vi "Sig2MS Process.vi"(5 "SigProc":bool, 6 "error in (no error)":errorcluster, 7 "Index":i32=-1, 8 "signal in":waveform(sgl), 9 "SkipIon":bool) -> (0 "error out":errorcluster, 1 "Ionisation signal out":waveform(sgl)[](array[waveform]), 2 "spectraData":waveform(sgl)[](array[waveform]), 4 "signalDataAttr":T1)   [LabVIEW 2018]
uses:
  Sig2MS.lvclass
  ctl/signalDataAttr.ctl
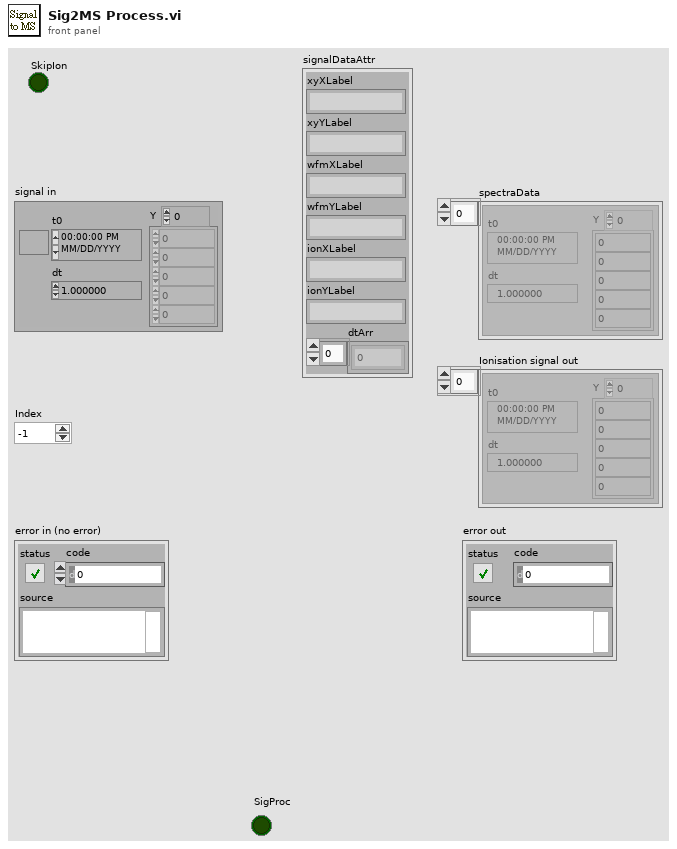
[diagram p1: front panel]
types:
  T1 = typedef "signalDataAttr.ctl" = cluster{"xyXLabel":string, "xyYLabel":string, "wfmXLabel":string, "wfmYLabel":string, "ionXLabel":string, "ionYLabel":string, "dtArr":dbl[]}
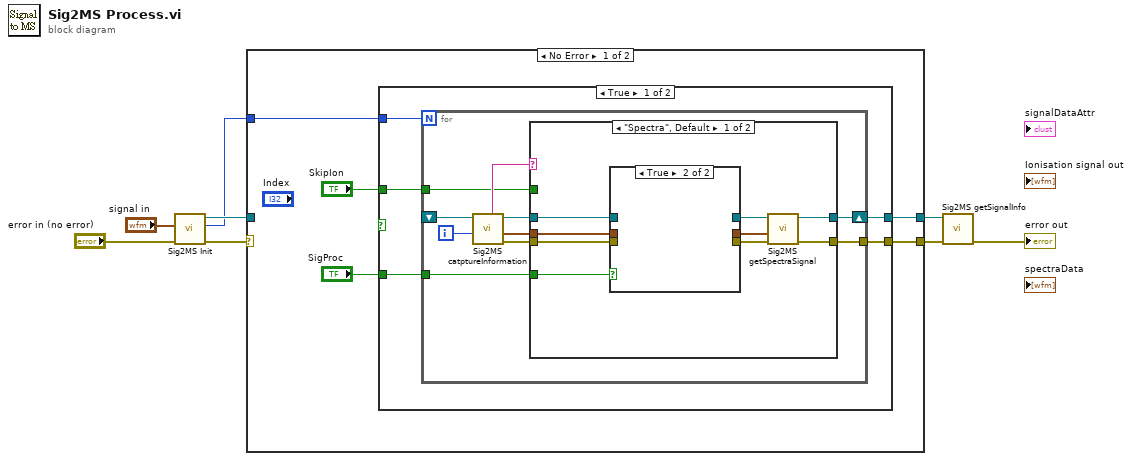
[diagram p0: block diagram]
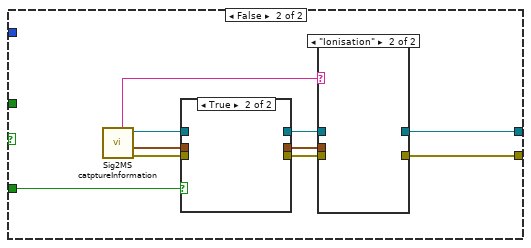
[diagram p5: hidden frame]
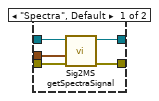
[diagram p7: hidden frame]
diagram:
  n1 = call "Sig2MS Init.vi"("error in (no error)"="error in (no error)", "signal in"="signal in") -> ("error out"=w5:errorcluster, "Size"=w2:i32, "Sig2MS out"=w6:refnum<class "Sig2MS.lvclass">)  [unwired: 7 in]
  n2 = case shown="No Error" w5 {
    selector: w5 -> [_ w68]
    tunnel: w6 -> [_ w69]
    tunnel: w2 -> [w13 _]
    tunnel: [w11 w68] -> w3
    tunnel: [w10 w69] -> w4
    frame No Error {
      n3 = case shown="True" {
        selector: _ -> [_ _]
        tunnel: w13 -> [w17 _]
        tunnel: "SigProc" -> [w18 w59]
        tunnel: [w16 w58] -> w11
        tunnel: [w15 w52] -> w10
        tunnel: "SkipIon" -> [w14 _]
        frame True {
          n4 = for {
            N: w17 -> [_]
            tunnel: w18 -> [w20]
            shift-right: [w27] -> w15
            shift-left: _ -> [w28]
            tunnel: [w26] -> w16
            tunnel: w14 -> [w19]
            i -> [w25]
            n5 = call "Sig2MS catptureInformation.vi"("Index"=w25, "Sig2MS in"=w28) -> ("error out"=w21:errorcluster, "SectionalSig"=w22:waveform(sgl), "Sig2MS out"=w23:refnum<class "Sig2MS.lvclass">, "Label"=w24:string)  [unwired: 6 in]
            n6 = case shown="\"Spectra\", Default" w24 {
              tunnel: w21 -> [w34 w43]
              tunnel: w23 -> [w36 w45]
              tunnel: w22 -> [w35 w44]
              tunnel: [w32 w47] -> w27
              tunnel: [w31 w46] -> w26
              tunnel: w20 -> [w37 w42]
              tunnel: w19 -> [_ w41]
              frame "Spectra", Default {
                n7 = case shown="True" w37 {
                  tunnel: w36 -> [w40 _]
                  tunnel: w34 -> [w39 _]
                  tunnel: [w39 _] -> w30
                  tunnel: [w40 _] -> w33
                  tunnel: w35 -> [w38 _]
                  tunnel: [w38 _] -> w29
                  frame False {
                  }
                  frame True {
                  }
                }
                n8 = call "Sig2MS getSpectraSignal.vi"("error in (no error)"=w30, "signal in"=w29, "Sig2MS in"=w33) -> ("error out"=w31:errorcluster, "Sig2MS out"=w32:refnum<class "Sig2MS.lvclass">)  [unwired: 7 in]
              }
              frame "Ionisation" {
                n9 = case shown="False" w41 {
                  tunnel: [_ w49] -> w47
                  tunnel: [_ w48] -> w46
                  tunnel: w45 -> [_ w49]
                  tunnel: w44 -> [_ _]
                  tunnel: w43 -> [_ w48]
                  tunnel: w42 -> [_ _]
                  frame False {
                  }
                  frame True {
                  }
                }
              }
            }
          }
        }
        frame False {
          n10 = call "Sig2MS catptureInformation.vi"() -> ("error out"=w56:errorcluster, "SectionalSig"=w50:waveform(sgl), "Sig2MS out"=w57:refnum<class "Sig2MS.lvclass">, "Label"=w51:string)  [unwired: 8 in]
          n11 = case shown="True" w59 {
            tunnel: w57 -> [w62 _]
            tunnel: w56 -> [w61 _]
            tunnel: [w61 _] -> w55
            tunnel: [w62 _] -> w54
            tunnel: w50 -> [w60 _]
            tunnel: [w60 _] -> w53
            frame False {
            }
            frame True {
            }
          }
          n12 = case shown="\"Ionisation\"" w51 {
            tunnel: w55 -> [w63 _]
            tunnel: w54 -> [w67 _]
            tunnel: w53 -> [w64 _]
            tunnel: [w66 _] -> w52
            tunnel: [w65 _] -> w58
            frame "Spectra", Default {
              n13 = call "Sig2MS getSpectraSignal.vi"("error in (no error)"=w63, "signal in"=w64, "Sig2MS in"=w67) -> ("error out"=w65:errorcluster, "Sig2MS out"=w66:refnum<class "Sig2MS.lvclass">)  [unwired: 7 in]
            }
            frame "Ionisation" {
            }
          }
        }
      }
    }
    frame Error {
    }
  }
  n14 = call "Sig2MS getSignalInfo.vi"("error in (no error)"=w3, "Sig2MS in"=w4) -> ("error out"=→"error out":errorcluster)  [unwired: 7 in, 2 out]
